vi "FIRMWARE_-_0.2.vi"() -> ()   [LabVIEW 2017]
uses:
  <vilib>/LabVIEW Interface for Arduino/Type Defs/Board Type.ctl
  <vilib>/LabVIEW Interface for Arduino/Type Defs/Connection Type.ctl
  <vilib>/LabVIEW Interface for Arduino/Type Defs/Pin Mode.ctl
  <vilib>/LabVIEW Interface for Arduino/LabVIEW Interface for Arduino.lvlib
panel:
  in  "PORTA":refnum<visa-resource-name>
  out "SOPRADOR":bool
  out "DESVIO":bool
  in  "STOP":bool
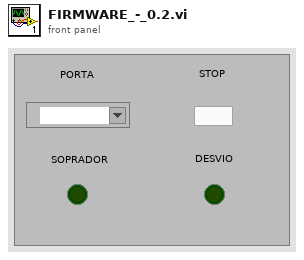
[diagram p1: front panel]
types:
  T1 = typedef "LabVIEW Interface for Arduino.lvlib/Connection Type.ctl" = enum8{"USB / Serial", "XBEE", "BlueSmirf (Bluetooth)"}
  T2 = typedef "LabVIEW Interface for Arduino.lvlib/Board Type.ctl" = enum16{"Uno", "Dimuelanove w/Atmega 328", "Mega 2560"}
  T3 = typedef "LabVIEW Interface for Arduino.lvlib/Arduino Resource.ctl" = cluster{"VISA resource":refnum<visa-resource-name>, "Board Type":T2, "Connection Type":enum8{"USB / Serial"}, "Bytes Per Packet (15)":u8}
  T4 = typedef "LabVIEW Interface for Arduino.lvlib/Pin Mode.ctl" = enum8{"Input", "Output"}
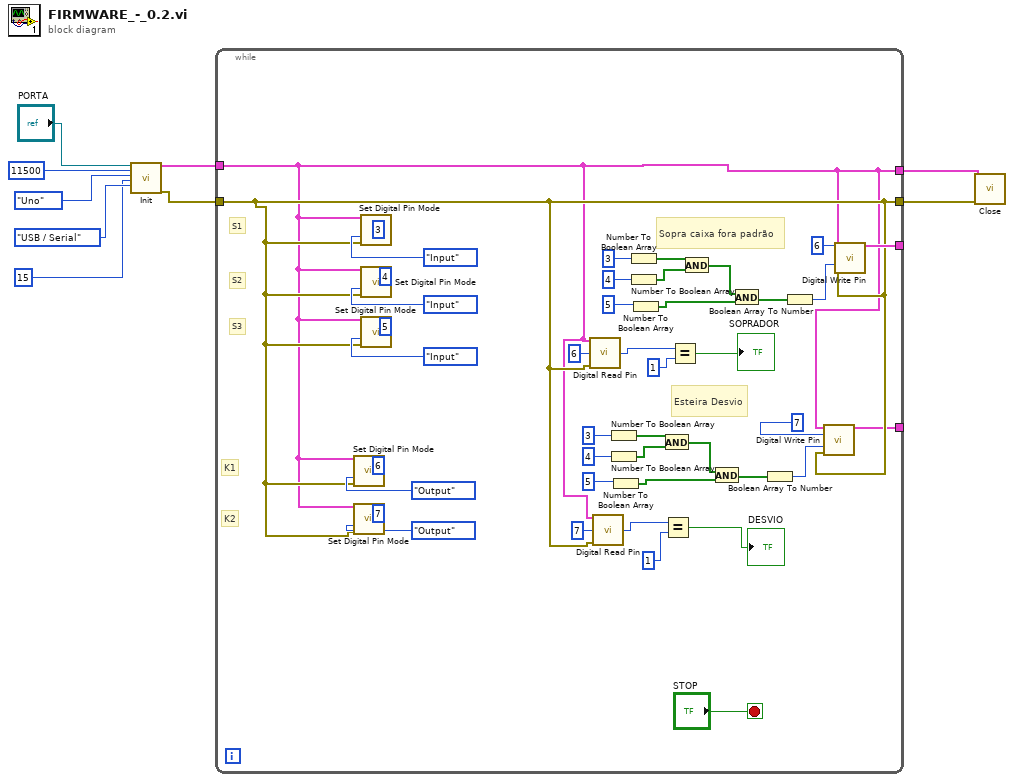
[diagram p0: block diagram]
diagram:
  n1 = call <vilib>:"Init.vi"("VISA resource"="PORTA", "Baud Rate (115200)"=u32 11500, "Board Type (Uno)"=Board_Type."Uno", "Bytes Per Packet (15)"=u32 15, "Connection Type (USB/Serial)"=Connection_Type."USB / Serial") -> ("Arduino Resource"=w9:T3, "error out"=w8:errorcluster)  [unwired: 13 in]
  n2 = while {
    tunnel: w9 -> [w14]
    tunnel: w8 -> [w15]
    tunnel: [w14] -> w2
    tunnel: [w15] -> w3
    tunnel: [w22] -> _
    tunnel: [w13] -> _
    stop <- "STOP" stop-if-true
    # "Esteira Desvio"
    # "Sopra caixa fora padrão"
    # "K2"
    # "K1"
    # "S3"
    # "S2"
    # "S1"
    n3 = call <vilib>:"Set Digital Pin Mode.vi"("Arduino Resource"=w14, "Digital I/O Pin"=u8 6, "Pin Mode (Input)"=Pin_Mode."Output", "error in"=w15) -> ()  [unwired: 10 in, 2 out]
    n4 = call <vilib>:"Set Digital Pin Mode.vi"("Arduino Resource"=w14, "Digital I/O Pin"=u8 7, "Pin Mode (Input)"=Pin_Mode."Output", "error in"=w15) -> ()  [unwired: 10 in, 2 out]
    n5 = call <vilib>:"Set Digital Pin Mode.vi"("Arduino Resource"=w14, "Digital I/O Pin"=u8 3, "Pin Mode (Input)"=Pin_Mode."Input", "error in"=w15) -> ()  [unwired: 10 in, 2 out]
    n6 = call <vilib>:"Set Digital Pin Mode.vi"("Arduino Resource"=w14, "Digital I/O Pin"=u8 4, "Pin Mode (Input)"=Pin_Mode."Input", "error in"=w15) -> ()  [unwired: 10 in, 2 out]
    n7 = call <vilib>:"Set Digital Pin Mode.vi"("Arduino Resource"=w14, "Digital I/O Pin"=u8 5, "Pin Mode (Input)"=Pin_Mode."Input", "error in"=w15) -> ()  [unwired: 10 in, 2 out]
    n8 = call <vilib>:"Digital Read Pin.vi"("Arduino Resource"=w14, "Digital I/O Pin (0)"=u8 6, "error in"=w15) -> ("Value"=w20:u8)  [unwired: 10 in, 2 out]
    n9 = call <vilib>:"Digital Read Pin.vi"("Arduino Resource"=w14, "Digital I/O Pin (0)"=u8 7, "error in"=w15) -> ("Value"=w17:u8)  [unwired: 10 in, 2 out]
    n10 = Number To Boolean Array(number=u32 3) -> (Boolean array=w33:bool[])
    n11 = Number To Boolean Array(number=u32 4) -> (Boolean array=w32:bool[])
    n12 = Number To Boolean Array(number=u32 5) -> (Boolean array=w25:bool[])
    n13 = Number To Boolean Array(number=u32 3) -> (Boolean array=w42:bool[])
    n14 = Number To Boolean Array(number=u32 4) -> (Boolean array=w41:bool[])
    n15 = Number To Boolean Array(number=u32 5) -> (Boolean array=w35:bool[])
    n16 = And(x=w33, y=w32) -> (x .and. y?=w27:bool[])
    n17 = Equal?(x=w17, y=u8 1) -> (x = y?=→"DESVIO":bool)
    n18 = Equal?(x=w20, y=u8 1) -> (x = y?=→"SOPRADOR":bool)
    n19 = And(x=w42, y=w41) -> (x .and. y?=w37:bool[])
    n20 = And(x=w27, y=w25) -> (x .and. y?=w26:bool[])
    n21 = And(x=w37, y=w35) -> (x .and. y?=w36:bool[])
    n22 = Boolean Array To Number(Boolean array=w26) -> (number=w29:u32)
    n23 = Boolean Array To Number(Boolean array=w36) -> (number=w38:u32)
    n24 = call <vilib>:"Digital Write Pin.vi"("Arduino Resource"=w14, "Digital I/O Pin (0)"=u8 7, "Value (0)"=w29, "error in"=w15) -> ("Arduino Resource"=w13:T3)  [unwired: 10 in, 1 out]
    n25 = call <vilib>:"Digital Write Pin.vi"("Arduino Resource"=w14, "Digital I/O Pin (0)"=u8 6, "Value (0)"=w38, "error in"=w15) -> ("Arduino Resource"=w22:T3)  [unwired: 10 in, 1 out]
  }
  n26 = call <vilib>:"Close.vi"("Arduino Resource"=w2, "error in"=w3) -> ()  [unwired: 13 in, 1 out]
